vi "Sr830 ReadCh.vi"(0 "VISA Rsrc":refnum<visa-resource-name>="SR830A", 1 "Autoscale":bool=TRUE, 5 "Channels":u16(ring) items=["X and Y", "R and Têta", "X, Y, R and Têta"], 7 "Délais":u32, 9 "Check Status":bool, 11 "error in (no error)":errorcluster, 12 "Ask Correction":bool, 13 "Show Warning":bool=TRUE caption="Show Warning\nMessage") -> (3 "Warning":bool, 4 "Ressource VISA Out":refnum<visa-resource-name>="GPIB0::8::INSTR", 6 "Outputs":dbl[](array[numeric]), 10 "Status Byte":bool[](array[boolean]), 14 "Ask Correction Out":bool, 15 "error out":errorcluster)   [LabVIEW 2019]
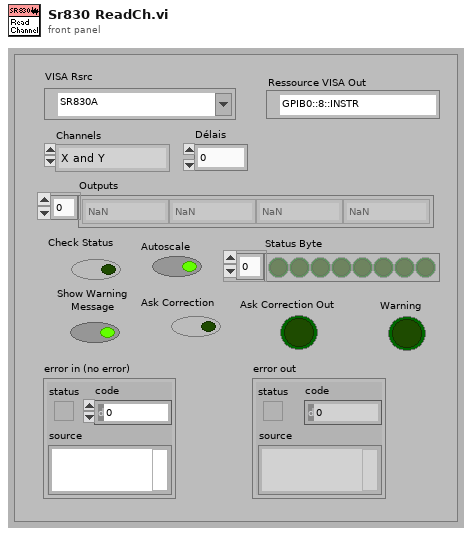
[diagram p1: front panel]
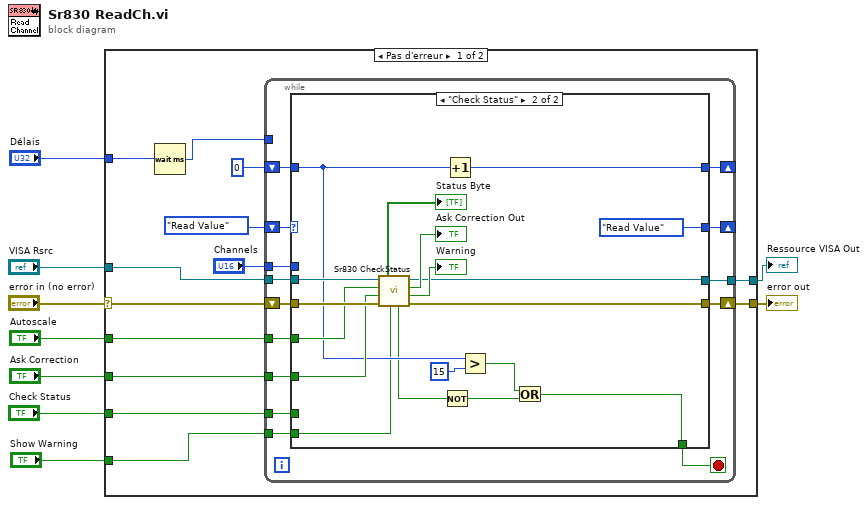
[diagram p0: block diagram]
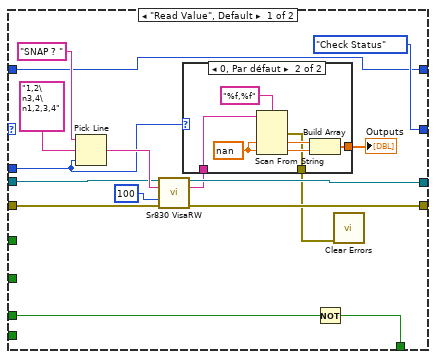
[diagram p2: hidden frame]
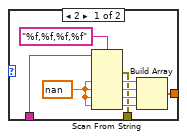
[diagram p3: hidden frame]
diagram:
  n1 = case shown="Pas d'erreur" "error in (no error)" {
    selector: "error in (no error)" -> [w15 w88]
    tunnel: [w21 w88] -> w8
    tunnel: "Autoscale" -> [w20 _]
    tunnel: "Check Status" -> [w17 _]
    tunnel: "VISA Rsrc" -> [w16 w87]
    tunnel: "Ask Correction" -> [w14 _]
    tunnel: [w13 w87] -> w3
    tunnel: "Délais" -> [w12 _]
    tunnel: "Show Warning" -> [w10 _]
    frame No Error {
      n2 = Wait (ms)(milliseconds to wait=w12) -> (millisecond timer value=w11:u32)
      n3 = while {
        shift-right: [w32] -> _
        shift-left: enum16{"Read Value", "Check Status"}."Read Value" -> [w36]
        shift-right: [w34] -> w21
        shift-left: w15 -> [w35]
        tunnel: w20 -> [w31]
        tunnel: "Channels" -> [w30]
        shift-right: [w28] -> _
        shift-left: 0 ("timeout ms (488.2 global)") -> [w29]
        tunnel: w17 -> [w27]
        tunnel: w16 -> [w26]
        tunnel: w14 -> [w25]
        tunnel: [w24] -> w13
        tunnel: w11 -> [_]
        tunnel: w10 -> [w23]
        stop <- w33 stop-if-true
        n4 = case shown="\"Check Status\"" w36 {
          tunnel: w35 -> [w51 w86]
          tunnel: [w42 w84] -> w34
          tunnel: [w45 w74] -> w33
          tunnel: [enum16{"Read Value", "Check Status"}."Check Status" enum16{"Read Value", "Check Status"}."Read Value"] -> w32
          tunnel: w31 -> [_ w82]
          tunnel: w30 -> [w40 _]
          tunnel: w29 -> [w38 w76]
          tunnel: [w38 w77] -> w28
          tunnel: w27 -> [w46 _]
          tunnel: w26 -> [w49 w85]
          tunnel: w25 -> [_ w79]
          tunnel: [w44 w72] -> w24
          tunnel: w23 -> [_ w69]
          frame "Read Value", Default {
            n5 = Pick Line(string ("")="SNAP ? " ("chaîne (\"\")"), multi-line string="1,2\n3,4\n1,2,3,4" ("data"), line index=w40) -> (output string=w50:string)
            n6 = call <userlib>:"Sr830 VisaRW.vi"("VISA Rsrc"=w49, "ChaineCom"=w50, "Nbcaract"=u32 100, "error in (no error)"=w51) -> ("VISA Rsrc Out"=w44:refnum<visa-resource-name>, "ChaineRep"=w43:string, "error out"=w42:errorcluster)  [unwired: 8 in, 1 out]
            n7 = case shown="0, Par défaut" w40 {
              tunnel: w43 -> [w61 w68]
              tunnel: [w55 w65] -> w39
              tunnel: [w53 w62] -> w37
              frame 2 {
                w60 = nan ("valeur par défaut 3")
                n8 = Scan From String(format string="%f,%f,%f,%f" ("chaîne de format"), input string=w61, default 1=w60, default 2=w60, default 3=w60, default 4=w60) -> (error out=w53:errorcluster, output 1=w56:dbl, output 2=w57:dbl, output 3=w58:dbl, output 4=w59:dbl)  [unwired: 2 in, 2 out]
                n9 = Build Array(w56, w57, w58, w59) -> (w55:dbl[])
              }
              frame 0, Default {
                w64 = nan ("valeur par défaut 1")
                n10 = Scan From String(format string="%f,%f" ("chaîne de format"), input string=w68, default 1=w64, default 2=w64) -> (error out=w62:errorcluster, output 1=w67:dbl, output 2=w66:dbl)  [unwired: 2 in, 2 out]
                n11 = Build Array(w67, w66) -> (w65:dbl[])
              }
            }
            "Outputs" <- w39
            n12 = Not(x=w46) -> (.not. x?=w45:bool)
            n13 = call <vilib>:"Clear Errors.vi"("error in (no error)"=w37) -> ()  [unwired: 5 in, 2 out]
          }
          frame "Check Status" {
            n14 = call <userlib>:"Sr830 CheckStatus.vi"("Show Warning"=w69, "error in (no error)"=w86, "Ask Correction"=w79, "Autoscale"=w82, "Ressource VISA In"=w85) -> ("error out"=w84:errorcluster, "Warning"=→"Warning":bool, "Ask Correction Out"=→"Ask Correction Out":bool, "Ressource VISA Out"=w72:refnum<visa-resource-name>, "Reprise"=w71:bool, "Status Byte"=→"Status Byte":bool[])
            n15 = Not(x=w71) -> (.not. x?=w70:bool)
            n16 = Increment(x=w76) -> (x+1=w77:i32)
            n17 = Greater?(x=w76, y=15) -> (0:w73:bool)
            n18 = Or(x=w73, y=w70) -> (x .or. y?=w74:bool)
          }
        }
      }
    }
    frame Error {
    }
  }
  "error out" <- w8
  "Ressource VISA Out" <- w3
